vi "2 PureWaypointHeadingGoodness.vi"(3 "Desired Heading":T1 format="%05.1f", 4 "Heading to Test":dbl) -> (1 "Goodness":dbl)   [LabVIEW 2011]
doc: "Takes the absolute wind vector, the heading of your next waypoint, and a test heading and outputs a goodness value for the test heading. The criteria is the speed to get to the waypoint.\n\nThe goodness is evaluated by taking the softmax of an angle with all possible complimenting angles (i.e. if the test heading is 10 degrees it is matched with -1 through -89; note that angles are adjusted to be degrees from directly at the waypoint). The specific calculation for finding the net velocity of a pair of angles requires the velocities from the polar plot."
uses:
  2 Typedefs/heading.ctl
panel:
  # "Inputs"
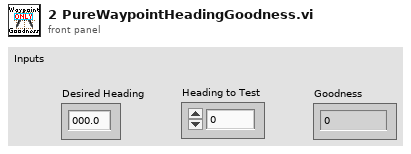
[diagram p1: front panel]
types:
  T1 = typedef "heading.ctl" = dbl
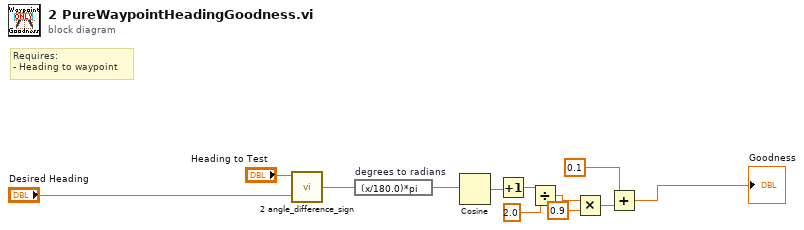
[diagram p0: block diagram]
diagram:
  # "Requires:\n- Heading to waypoint"
  n1 = call "2 angle_difference_sign.vi"("Angle 2"="Desired Heading", "Angle 1"="Heading to Test") -> ("Difference"=w10:dbl)
  n2 = expression code="(x/180.0)*pi" "degrees to radians"(w10) -> (w11:dbl)
  n3 = Cosine(x=w11) -> (cos(x)=w9:dbl)
  n4 = Increment(x=w9) -> (x+1=w8:dbl)
  n5 = Divide(x=w8, y=2.0) -> (x/y=w6:dbl)
  n6 = Multiply(x=w6, y=0.9) -> (x*y=w4:dbl)
  n7 = Add(x=0.1, y=w4) -> (x+y=→"Goodness":dbl)
